vi "SetParam.vi"(8 "error in (no error)":errorcluster caption="entrée d'erreur (pas d'erreur)", 10 "minmax_scale":T1={"feature_range"={"min"=0.0, "max"=1.0}, "axis"=0, "copy"=TRUE}, 11 "minmax_scale.lvclass":refnum<class "minmax_scale.lvclass">) -> (0 "error out":errorcluster caption="sortie d'erreur", 3 "minmax_scale.lvclass":refnum<class "minmax_scale.lvclass">)   [LabVIEW 2020, in "minmax_scale.lvclass"]
doc: "Set Parameters"
uses:
  minmax_scale.lvclass
  minmax_scale.lvclass/minmax_scale.ctl
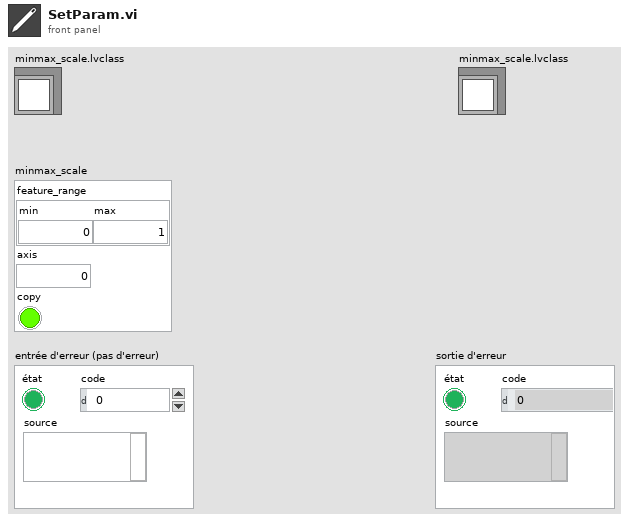
[diagram p1: front panel]
types:
  T1 = cluster{"feature_range":cluster{"min":dbl, "max":dbl}, "axis":i32, "copy":bool}
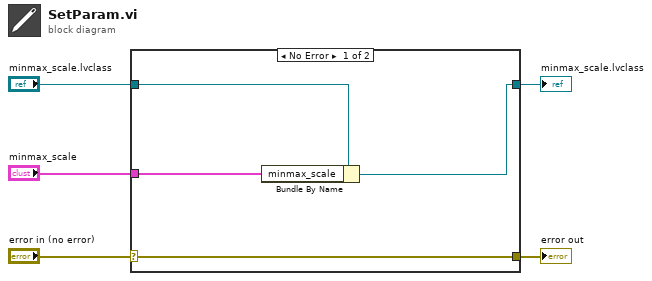
[diagram p0: block diagram]
diagram:
  n1 = case shown="No Error" "error in (no error)" {
    selector: "error in (no error)" -> [w9 w10]
    tunnel: [w9 w10] -> w4
    tunnel: [w7 w11] -> w2
    tunnel: "minmax_scale.lvclass" -> [w8 w11]
    tunnel: "minmax_scale" -> [w6 _]
    frame No Error {
      n2 = Bundle By Name(cluster=w8, "minmax_scale"=w6) -> (w7:refnum<class "minmax_scale.lvclass">)
    }
    frame Error {
    }
  }
  "error out" <- w4
  "minmax_scale.lvclass" <- w2
